vi "write_data.vi"(8 "error in (no error)":errorcluster, 10 "data":T1, 11 "BayesianRidge in":refnum<class "BayesianRidge.lvclass">) -> (0 "error out":errorcluster, 3 "BayesianRidge out":refnum<class "BayesianRidge.lvclass">)   [LabVIEW 2020, in "BayesianRidge.lvclass"]
uses:
  BayesianRidge.lvclass
  Controls/bayesian_ridge_data.ctl
  BayesianRidge.lvclass/BayesianRidge.ctl
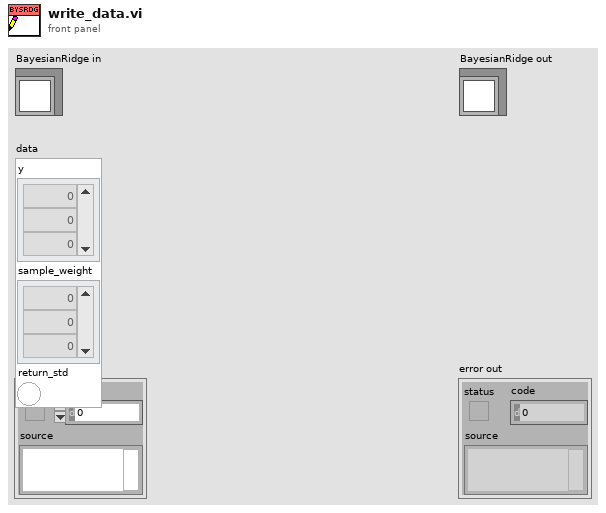
[diagram p1: front panel]
types:
  T1 = typedef "bayesian_ridge_data.ctl" = cluster{"y":dbl[][], "sample_weight":dbl[], "return_std":bool}
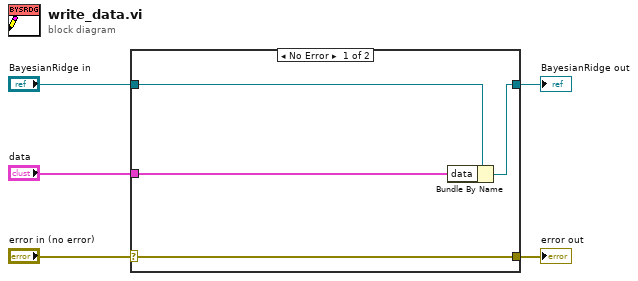
[diagram p0: block diagram]
diagram:
  n1 = case shown="No Error" "error in (no error)" {
    selector: "error in (no error)" -> [w9 w10]
    tunnel: [w9 w10] -> w4
    tunnel: [w7 w11] -> w2
    tunnel: "BayesianRidge in" -> [w8 w11]
    tunnel: "data" -> [w6 _]
    frame No Error {
      n2 = Bundle By Name(cluster=w8, "data"=w6) -> (w7:refnum<class "BayesianRidge.lvclass">)
    }
    frame Error {
    }
  }
  "error out" <- w4
  "BayesianRidge out" <- w2
